vi "SettleDrift.vi"() -> ()   [LabVIEW 2021]
uses:
  shared/CorrelImages (SubVI)Single.vi
  <userlib>/Nanonis Prog Interface V5/Nanonis Prog Interface.lvlib
panel:
  out "Saturation status":T1
  out "Compensation speeds (m/s)":cluster{"Vx":sgl, "Vy":sgl, "Vz":sgl} {"Vz" format="%#_5p"; "Vy" format="%#_5p"; "Vx" format="%#_5p"}
  out "Compensation status":bool
  in  "active drift compensation":bool
  out "y drift/sec":sgl format="%#_6p"
  out "x drift/sec":sgl format="%#_6p"
  out "seconds per image":dbl
  out "loops":i32
  in  "stop":bool
  out "x drift":sgl format="%#_6p"
  out "y drift":sgl format="%#_6p"
  out "y Drift":sgl(graph)
  out "X Drift":sgl(graph)
  in  "Drift correction Pixels":i32=256
  in  "Img Current":sgl=1e-11 format="%#_6p"
  in  "Img Bias (V)":sgl=-0.002 format="%_2p"
  in  "Img Speed":sgl=1.5e-07 format="%#_6p"
  in  "Channel index (0-23)":u8(ring) items=["Current"=0, "Z (m)"=14]
  # "Turn continuous scan off\ndo not use june 2017!"
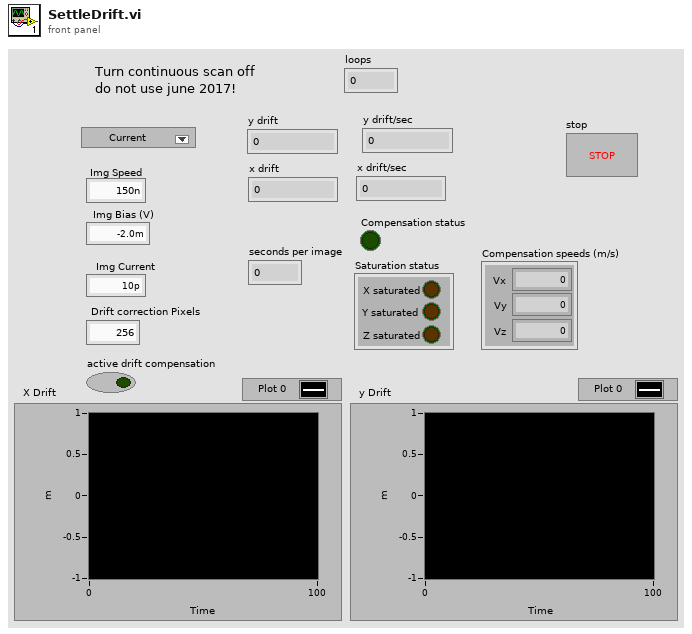
[diagram p1: front panel]
types:
  T1 = cluster{"X saturated":bool, "Y saturated":bool, "Z saturated":bool}
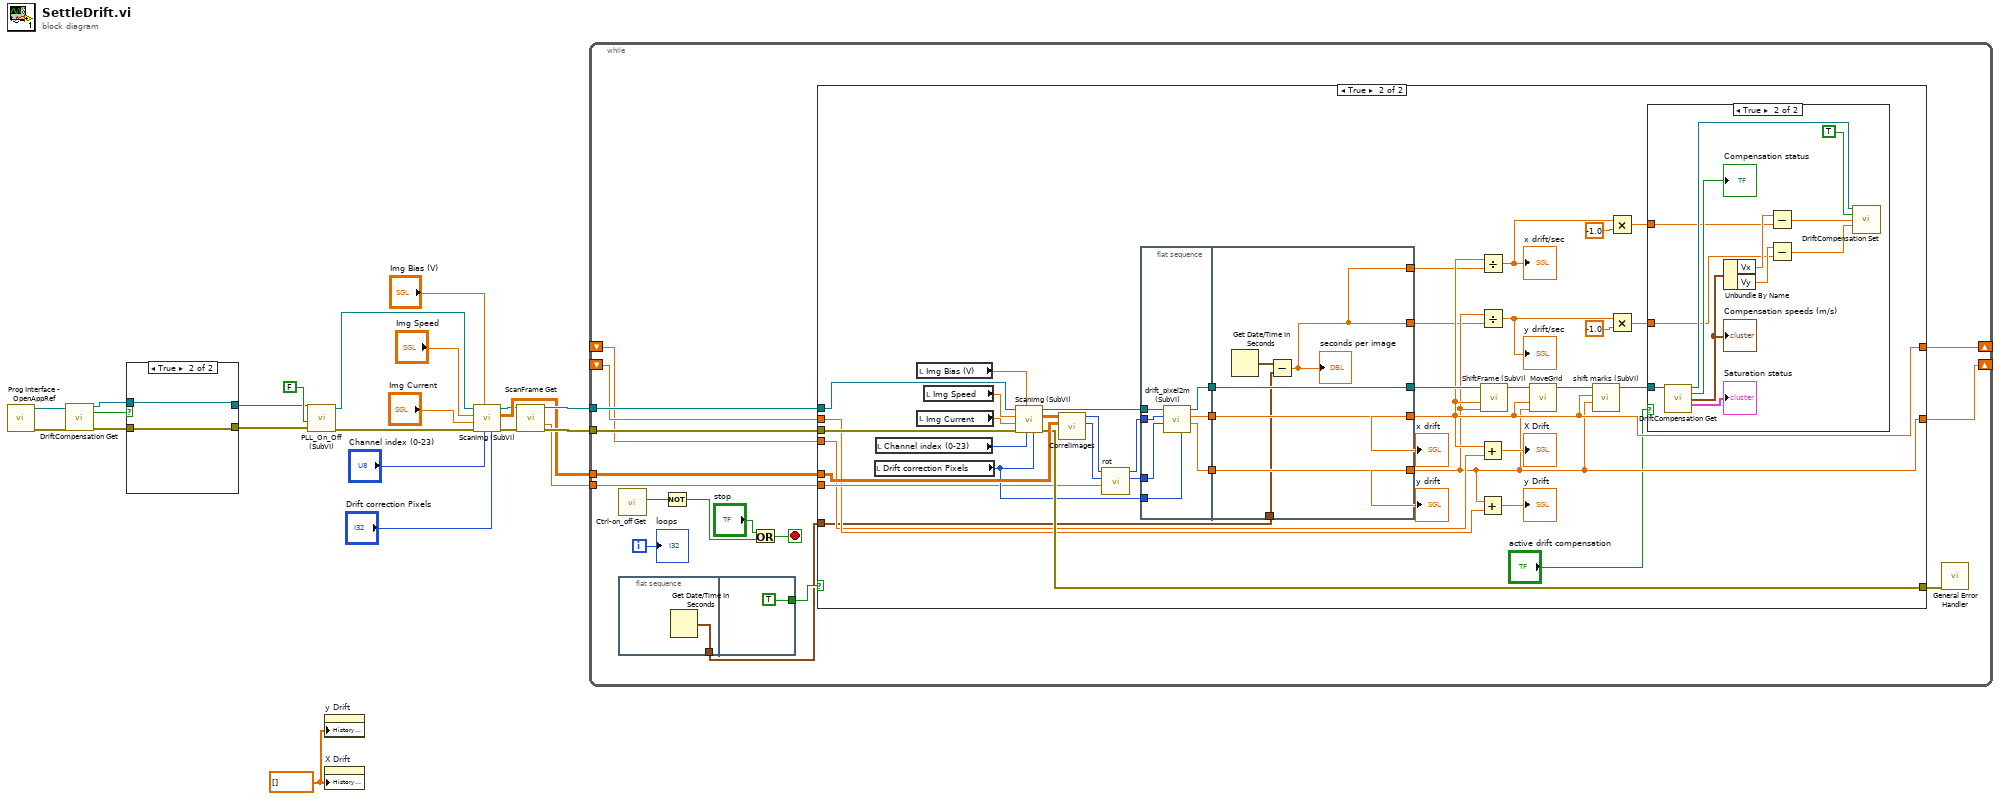
[diagram p0: block diagram]
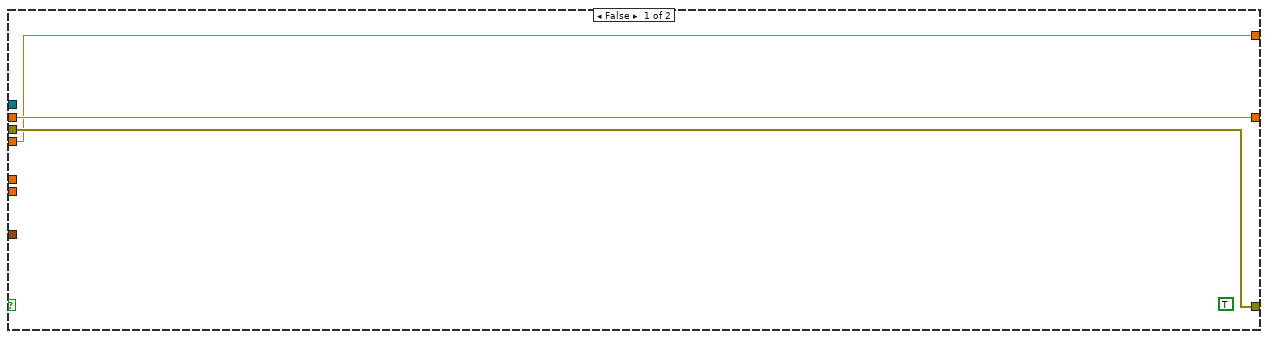
[diagram p2: hidden frame]
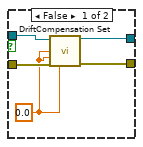
[diagram p4: hidden frame]
diagram:
  w8 = sgl[] [] ("History Data")
  n1 = call <userlib>:"Prog Interface - OpenAppRef.vi"() -> ("Error out"=w6:errorcluster, "Application reference"=w7:refnum<vi>)  [unwired: 6 in]
  n2 = call <userlib>:"DriftCompensation Get.vi"("Application ref in"=w7, "error in (no error)"=w6) -> ("Application ref out"=w4:refnum<vi>, "Compensation status"=w5:bool, "error out"=w3:errorcluster)  [unwired: 9 in, 2 out]
  n3 = case shown="True" w5 {
    tunnel: w4 -> [w27 w29]
    tunnel: w3 -> [w26 w28]
    tunnel: [w24 w29] -> w2
    tunnel: [w23 w28] -> w1
    frame False {
      w25 = sgl 0.0 ("Vx (m/s)")
      n4 = call <userlib>:"DriftCompensation Set.vi"("Application ref in"=w27, "Vx (m/s)"=w25, "Vy (m/s)"=w25, "error in (no error)"=w26, "Vz (m/s)"=w25) -> ("Application ref out"=w24:refnum<vi>, "error out"=w23:errorcluster)  [unwired: 9 in]
    }
    frame True {
    }
  }
  n5 = call "PLL_On_Off (SubVI).vi"("error in (no error)"=w1, "Output ON/OFF (F=OFF)"=FALSE, "Application in"=w2) -> ("error out"=w13:errorcluster, "Application out"=w14:refnum<vi>)  [unwired: 7 in]
  n6 = property on="y Drift" class="WFChart (strict)"("History Data"=w8) -> ()  [unwired: 2 in, 2 out]
  n7 = property on="X Drift" class="WFChart (strict)"("History Data"=w8) -> ()  [unwired: 2 in, 2 out]
  n8 = call "ScanImg (SubVI).vi"("pixel"="Drift correction Pixels", "Channel index (0-23)"="Channel index (0-23)", "Bias (V)"="Img Bias (V)", "error in (no error)"=w13, "Current"="Img Current", "Img Speed"="Img Speed", "Application in"=w14) -> ("error out"=w9:errorcluster, "Img"=w20:dbl[][], "Application out"=w10:refnum<vi>)  [unwired: 2 in]
  n9 = call <userlib>:"ScanFrame Get.vi"("Application ref in"=w10, "error in (no error)"=w9) -> ("Application ref out"=w22:refnum<vi>, "Angle (deg)"=w19:sgl, "error out"=w21:errorcluster)  [unwired: 9 in, 2 out]
  n10 = while {
    tunnel: w22 -> [w45]
    tunnel: w21 -> [w44]
    tunnel: w20 -> [w43]
    tunnel: w19 -> [w42]
    shift-right: [w39] -> _
    shift-left: _ -> [w38]
    shift-right: [w40] -> _
    shift-left: _ -> [w37]
    i -> [w33]
    stop <- w36 stop-if-true
    n11 = call <userlib>:"Ctrl-on_off Get.vi"() -> ("Z-Controller on/off status"=w35:bool)  [unwired: 9 in, 2 out]
    n12 = flat-sequence {
      tunnel: [w46] -> w30
      tunnel: [TRUE] -> w31
      frame #0 {
        n13 = Get Date/Time In Seconds() -> (seconds since 1Jan1904=w46:timestamp)
      }
      frame #1 {
      }
    }
    n14 = Not(x=w35) -> (.not. x?=w34:bool)
    n15 = Or(x="stop", y=w34) -> (x .or. y?=w36:bool)
    n16 = case shown="True" w31 {
      tunnel: w43 -> [_ w89]
      tunnel: w45 -> [_ w73]
      tunnel: w44 -> [w50 w88]
      tunnel: [w50 w87] -> w32
      tunnel: w42 -> [_ w78]
      tunnel: [w48 w62] -> w40
      tunnel: [w49 w60] -> w39
      tunnel: w38 -> [w49 w68]
      tunnel: w37 -> [w48 w67]
      tunnel: w30 -> [_ w63]
      frame False {
        (unwired) TRUE ("DC active")
      }
      frame True {
        n17 = local read "Drift correction Pixels"() -> (w79:i32)
        n18 = local read "Channel index (0-23)"() -> (w82:u8)
        n19 = local read "Img Bias (V)"() -> (w83:sgl)
        n20 = local read "Img Current"() -> (w84:sgl)
        n21 = local read "Img Speed"() -> (w85:sgl)
        n22 = call "ScanImg (SubVI).vi"("pixel"=w79, "Channel index (0-23)"=w82, "Bias (V)"=w83, "error in (no error)"=w88, "Current"=w84, "Img Speed"=w85, "Application in"=w73) -> ("error out"=w87:errorcluster, "Img"=w86:dbl[][], "Application out"=w80:refnum<vi>)  [unwired: 2 in]
        n23 = call-poly "CorrelImages.vi"("Ref Array"=w89, "New Image"=w86) -> ("Y drift"=w75:i32, "X drift"=w77:i32)  [unwired: 6 in, 2 out]
        n24 = call "rot.vi"("angle"=w78, "y"=w75, "x"=w77) -> ("y'"=w74:i32, "x'"=w76:i32)  [unwired: 7 in]
        n25 = flat-sequence {
          tunnel: w80 -> [w107]
          tunnel: w79 -> [w106]
          tunnel: w76 -> [w105]
          tunnel: w74 -> [w104]
          tunnel: [w108] -> w66
          tunnel: [w103] -> w65
          tunnel: [w102] -> w64
          tunnel: [w112] -> w60
          tunnel: [w113] -> w62
          tunnel: [w114] -> w81
          tunnel: w66 -> [w114]
          tunnel: w65 -> [w113]
          tunnel: w64 -> [w112]
          tunnel: w63 -> [w110]
          tunnel: [w109] -> w61
          tunnel: [w109] -> w59
          frame #0 {
            n26 = call "drift_pixel2m (SubVI).vi"("Application in"=w107, "X drift"=w105, "Y drift"=w104, "Drift correction Pixels"=w106) -> ("Application out"=w108:refnum<vi>, "x drift"=w103:sgl, "y drift"=w102:sgl)  [unwired: 2 in, 1 out]
          }
          frame #1 {
            n27 = Get Date/Time In Seconds() -> (seconds since 1Jan1904=w111:timestamp)
            n28 = Subtract(x=w111, y=w110) -> (x-y=w109:dbl)
            "seconds per image" <- w109
          }
        }
        n29 = Add(x=w62, y=w67) -> (x+y=→"X Drift":sgl)
        n30 = Add(x=w60, y=w68) -> (x+y=→"y Drift":sgl)
        n31 = Divide(x=w62, y=w61) -> (x/y=w55:dbl)
        "x drift/sec" <- w55
        n32 = Divide(x=w60, y=w59) -> (x/y=w56:dbl)
        "y drift/sec" <- w56
        n33 = call "ShiftFrame (SubVI).vi"("Y shift"=w60, "X shift"=w62, "Application in"=w81) -> ("Application out"=w72:refnum<vi>)  [unwired: 8 in]
        n34 = call "MoveGrid.vi"("y"=w60, "x"=w62, "Application ref in"=w72) -> ("Application ref out"=w71:refnum<vi>)  [unwired: 7 in, 1 out]
        n35 = call "shift marks (SubVI).vi"("y"=w60, "x"=w62, "Application in"=w71) -> ("Application out"=w57:refnum<vi>)  [unwired: 7 in, 1 out]
        n36 = Multiply(x=w55, y=-1.0) -> (x*y=w53:dbl)
        n37 = Multiply(x=w56, y=-1.0) -> (x*y=w54:dbl)
        n38 = case shown="True" "active drift compensation" {
          tunnel: w57 -> [_ w101]
          tunnel: w54 -> [_ w93]
          tunnel: w53 -> [_ w92]
          frame False {
          }
          frame True {
            n39 = call <userlib>:"DriftCompensation Get.vi"("Application ref in"=w101) -> ("Application ref out"=w100:refnum<vi>, "Compensation status"=→"Compensation status":bool, "Compensation speeds (m/s)"=w96:cluster{"Vx":sgl, "Vy":sgl, "Vz":sgl}, "Saturation status"=→"Saturation status":T1)  [unwired: 10 in, 1 out]
            "Compensation speeds (m/s)" <- w96
            n40 = Unbundle By Name(w96) -> ("Vx"=w95:sgl, "Vy"=w94:sgl)
            n41 = Subtract(x=w95, y=w92) -> (x-y=w91:dbl)
            n42 = Subtract(x=w94, y=w93) -> (x-y=w90:dbl)
            n43 = call <userlib>:"DriftCompensation Set.vi"("Application ref in"=w100, "Compensation On/Off"=TRUE, "Vx (m/s)"=w91, "Vy (m/s)"=w90) -> ()  [unwired: 10 in, 2 out]
          }
        }
        "y drift" <- w60
        "x drift" <- w62
      }
    }
    n44 = call <vilib>:"General Error Handler.vi"("error in (no error)"=w32) -> ()  [unwired: 10 in, 5 out]
    "loops" <- w33
  }
